vi "globalTearDown.vi"(8 "error in (no error)":errorcluster, 11 "Test_Blob in":refnum<class "Test_Queue.lvclass">) -> (0 "error out":errorcluster, 3 "Test_Blob out":refnum<class "Test_Queue.lvclass">)   [LabVIEW 2015, in "Test_Queue.lvclass"]
uses:
  Test_Queue.lvclass
  Global Parameters.vi
  <vilib>/addons/_JKI Toolkits/VI Tester/TestCase.llb/TestCase.lvclass
  Core/Session/Session.lvclass
  Queue/NI_Azure_Queue.lvlib
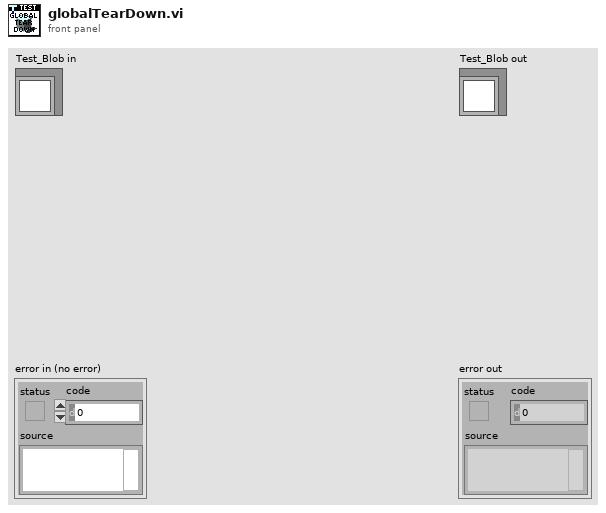
[diagram p1: front panel]
types:
  T1 = typedef "NI_Azure_Core.lvlib/Session.lvclass/Azure Credentials.ctl" = cluster{"Storage Account Name":string, "Access Key":string}
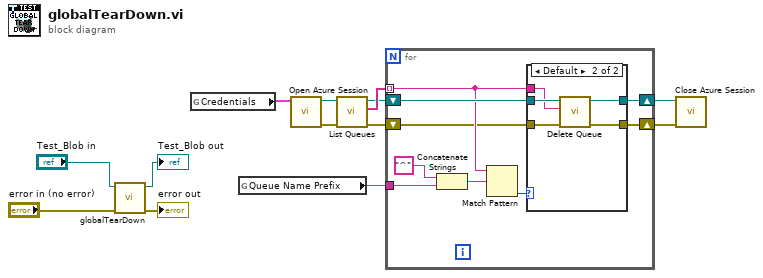
[diagram p0: block diagram]
diagram:
  n1 = call-parent "globalTearDown.vi"("error in (no error)"="error in (no error)", "TestCase in"="Test_Blob in") -> ("error out"=→"error out":errorcluster, "TestCase out"=→"Test_Blob out":refnum<class "Test_Queue.lvclass">)  [unwired: 8 in]
  n2 = global read "Global Parameters.vi" "Credentials"() -> (w8:T1)
  n3 = global read "Global Parameters.vi" "Queue Name Prefix"() -> (w5:string)
  n4 = call "Open Azure Session.vi"("Credentials"=w8) -> ("error out"=w4:errorcluster, "Azure Session"=w9:refnum<class "Session.lvclass">)  [unwired: 9 in]
  n5 = call "List Queues.vi"("error in (no error)"=w4, "Azure Session in"=w9) -> ("error out"=w3:errorcluster, "Queues"=w7:string[], "Azure Session out"=w6:refnum<class "Session.lvclass">)  [unwired: 7 in]
  n6 = for {
    tunnel: w7 -> [w17] mode=indexing
    tunnel: w5 -> [w20]
    shift-right: [w15] -> w2
    shift-left: w3 -> [w16]
    shift-right: [w14] -> w1
    shift-left: w6 -> [w19]
    n7 = Concatenate Strings("^" ("string"), w20) -> (w21:string)
    n8 = Match Pattern(string=w17, regular expression=w21) -> (offset past match=w18:i32)  [unwired: 1 in, 3 out]
    n9 = case shown="Default" w18 {
      tunnel: w19 -> [w23 w29]
      tunnel: w17 -> [_ w28]
      tunnel: w16 -> [w24 w27]
      tunnel: [w24 w26] -> w15
      tunnel: [w23 w25] -> w14
      frame -1 {
      }
      frame Default {
        n10 = call "Delete Queue.vi"("error in (no error)"=w27, "Queue"=w28, "Azure Session in"=w29) -> ("error out"=w26:errorcluster, "Azure Session out"=w25:refnum<class "Session.lvclass">)  [unwired: 7 in]
      }
    }
  }
  n11 = call "Close Azure Session.vi"("error in (no error)"=w2, "Azure Session"=w1) -> ()  [unwired: 9 in, 1 out]
